vi "Engine Control RT.vi"() -> ()   [LabVIEW 2015]
uses:
  <vilib>/Platform/TimedLoop/XDataNode/timing_clust.ctl
  <vilib>/Platform/TimedLoop/XDataNode/nitl_modes.ctl
  <vilib>/Platform/TimedLoop/XDataNode/wakeup.ctl
  <vilib>/FPGAPlugInAG/cRIO-9118/niLvFpga_Open_cRIO-9118.vi
  <vilib>/rvi/interface/common/dynamic/niFpgaDynamicAddResources.vi
  <vilib>/Utility/error.llb/Error Cluster From Error Code.vi
  <vilib>/rvi/errors/niLvFpgaAdjustHostInterfaceError.vi
  <vilib>/FPGAPlugInAG/Dynamic/niLvFpga_Close_Dynamic.vi
  <vilib>/Platform/TimedLoop/XDataNode/XDataNode.xnode
  <vilib>/rvi/interface/nirviOpenFPGA/nirviOpenFPGA.xnode
  FPGA Bitfiles/EngineControl.lvbitx
  <vilib>/rvi/interface/nirviReadWriteControl/nirviReadWriteControl.xnode
  <vilib>/rvi/interface/nirviCloseFPGA/nirviCloseFPGA.xnode
  <vilib>/Platform/TimedLoop/XDataNode/XDNodeRunTimeDep.lvlib
  <vilib>/rvi/interface/Simulation/niFpgaSimulationCallBeginRW.vi
  NiFpgaLv.dll
panel:
  in  "Tab Control":T1(tab)
  in  "SyncEnable":bool
  in  "SimEnable":bool
  in  "SimSpeed (RPM)":sgl=1000.0
  out "EngineSpeed (RPM)":sgl
  in  "EPTErrorClr":bool
  in  "TDC1 (CAD)":sgl
  out "MAX_CAT":u16=11520
  in  "Stroke (FALSE=2, TRUE=4)":bool=TRUE
  in  "NumberOfCrankTeeth":u16=360
  out "CrankStalled":bool=TRUE
  out "SyncStopped":bool=TRUE
  out "MissedCrankFlag":bool
  out "MissedCamFlag":bool
  out "CrankCount":u16 format="%02.0f"
  out "CAD":sgl format="%05.1f"
  in  "DIControl":T2={"ModuleEnable"=FALSE, "HVEnable"=FALSE, "InjectEnable"=FALSE, "Phase1FirstPeakEnable"=FALSE, "PiezoEnable"=FALSE, "PiezoInvert"=FALSE, "OneShotSelect"=enum."DISABLED", "One Shot Time (msec)"=1.0, "OneShot"=FALSE, "Fault_ClrSig"=FALSE, "HVTarget (V)"=75.0, "Back Boost Time (msec)"=0.25, "DI Scope Trigger Event"=0, "DI Scope Channel 2"=0} {"DI Scope Trigger Event" items=["INJECTION PULSE", "POWER SUPPLY ENABLED"]; "DI Scope Channel 2" items=["INTERNAL HIGH VOLTAGE", "EXTERNAL HIGH VOLTAGE", "BATTERY VOLTAGE"]}
  out "DIData":T3={"ModulePresent"=FALSE, "Module Temperature (C)"=0.0, "Internal High Voltage (V)"=0.0, "External High Voltage (V)"=0.0, "Battery Voltage (V)"=0.0, "Hardware Rev"="\u0000", "Firmware Rev"=0} {"Module Temperature (C)" format="%#.1g"; "Internal High Voltage (V)" format="%#.1f"; "External High Voltage (V)" format="%0#.1g"; "Battery Voltage (V)" format="%#.1g"}
  in  "Channel1 Enable":bool
  out "Critical Faults":T4
  out "Non Critical Faults":T5
  in  "PlsGen_Config":T6={"Window_Start (DBTDC)"=60.0, "Window_End (DBTDC)"=-60.0, "Enable_Inj1"=TRUE, "Duration_Inj1 (msec)"=1.0, "Timing_Inj1 (DBTDC)"=0.0, "Enable_Inj2"=FALSE, "Duration_Inj2 (msec)"=0.0, "Timing_Inj2 (DBTDC)"=0.0, "Enable_Inj3"=FALSE, "Duration_Inj3 (msec)"=0.0, "Timing_Inj3 (DBTDC)"=0.0, "Enable_Inj4"=FALSE, "Duration_Inj4 (msec)"=0.0, "Timing_Inj4 (DBTDC)"=0.0, "Enable_Inj5"=FALSE, "Duration_Inj5 (msec)"=0.0, "Timing_Inj5 (DBTDC)"=0.0}
  in  "DI IPhaseArrayIn":T7(array[cluster])=[{"DriveSrc"=TRUE, "IUpper (A)"=27.0, "ILower (A)"=26.0, "Dur (msec)"=0.3}, {"DriveSrc"=FALSE, "IUpper (A)"=15.0, "ILower (A)"=14.0, "Dur (msec)"=0.0}, {"DriveSrc"=FALSE, "IUpper (A)"=0.0, "ILower (A)"=0.0, "Dur (msec)"=0.0}, {"DriveSrc"=FALSE, "IUpper (A)"=0.0, "ILower (A)"=0.0, "Dur (msec)"=0.0}, {"DriveSrc"=FALSE, "IUpper (A)"=0.0, "ILower (A)"=0.0, "Dur (msec)"=0.0}, {"DriveSrc"=FALSE, "IUpper (A)"=0.0, "ILower (A)"=0.0, "Dur (msec)"=0.0}, {"DriveSrc"=FALSE, "IUpper (A)"=0.0, "ILower (A)"=0.0, "Dur (msec)"=0.0}, {"DriveSrc"=FALSE, "IUpper (A)"=0.0, "ILower (A)"=0.0, "Dur (msec)"=0.0}]
  in  "DIScopeRefresh":bool
  out "DIScope":cluster{sgl, sgl, sgl[][]}(graph)={-3.7e-05, 7.5e-06, array2x4500[9000 elements]}
  out "OLIntegrator":u32
  in  "PFIControl":T8={"ModuleEnable"=FALSE, "LS1Enable"=FALSE, "LS2Enable"=FALSE, "LS3Enable"=FALSE, "LS4Enable"=FALSE, "PFI1Enable"=FALSE, "PFI2Enable"=FALSE, "PFI3Enable"=FALSE, "PFI4Enable"=FALSE, "RecircAlways1"=FALSE, "RecircAlways2"=FALSE, "RecircAlways3"=FALSE, "RecircAlways4"=FALSE, "Phase1FirstPeak1"=FALSE, "Phase1FirstPeak2"=FALSE, "Phase1FirstPeak3"=FALSE, "Phase1FirstPeak4"=FALSE, "OneShotSelect"=enum."DISABLED", "One Shot Time (msec)"=5.0, "OneShot"=FALSE, "Fault_ClrSig"=FALSE}
  in  "PFI IPhaseArrayIn":cluster{"ISetpoint (A)":sgl, "Dur (msec)":sgl}[](array[cluster])=[{"ISetpoint (A)"=4.0, "Dur (msec)"=2.0}, {"ISetpoint (A)"=1.0, "Dur (msec)"=0.0}, {"ISetpoint (A)"=4.0, "Dur (msec)"=2.0}, {"ISetpoint (A)"=1.0, "Dur (msec)"=0.0}, {"ISetpoint (A)"=4.0, "Dur (msec)"=2.0}, {"ISetpoint (A)"=1.0, "Dur (msec)"=0.0}, {"ISetpoint (A)"=4.0, "Dur (msec)"=2.0}, {"ISetpoint (A)"=1.0, "Dur (msec)"=0.0}]
  out "PFIData":T9={"ModulePresent"=FALSE, "Hardware Rev"="\u0000", "Firmware Rev"=0}
  out "Critical Faults 2":T10
  out "Non Critical Faults 2":T11
  in  "LS4Duty":sgl=50.0
  in  "LS3Duty":sgl=50.0
  in  "LS2Duty":sgl=50.0
  in  "LS1Duty":sgl=50.0
  in  "LS4Freq":sgl=5.0
  in  "LS3Freq":sgl=5.0
  in  "LS2Freq":sgl=5.0
  in  "LS1Freq":sgl=5.0
  in  "FuelEnable2":bool
  in  "PFIDuration":sgl=4.0
  in  "CutoffPosition (DBTDC)":sgl=-180.0
  in  "TDC2":sgl=180.0
  in  "FuelTiming (DBTDC)":sgl
  in  "TDC1":sgl
  in  "FuelEnable1":bool
  in  "AfterDuration (msec)":sgl=15.0
  in  "AfterDelay (msec)":sgl=15.0
  in  "MainDuration (msec)":sgl=15.0
  in  "PilotDuration (msec)":sgl=15.0
  in  "PilotAdvance (msec)":sgl=15.0
  in  "AfterEnable1":bool
  in  "PilotEnable1":bool
  in  "MainEnable1":bool
  in  "Cutoff4 (DBTDC)":sgl
  in  "Cutoff3 (DBTDC)":sgl
  in  "Cutoff2 (DBTDC)":sgl
  in  "Cutoff1 (DBTDC)":sgl
  in  "MainSOI (DBTDC)":sgl
  in  "TDC (Absolute CAD)":sgl
  in  "SparkMaxDwell (msec)":sgl=15.0
  in  "SparkMinDwell (msec)":sgl=1.0
  in  "SparkDwell (msec)":sgl=3.0
  in  "SparkCutoffPosition (DBTDC)":sgl=-360.0
  in  "SparkEnd (DBTDC)":sgl
  in  "SparkStart (DBTDC)":sgl
  in  "FuelDuration (msec)":sgl=3.0
  in  "FuelCutoffPosition (DBTDC)":sgl=-360.0
  in  "FuelEnd (DBTDC)":sgl
  in  "FuelStart (DBTDC)":sgl
  in  "SparkActiveLow":bool
  in  "SparkPositionMode (F=End, T=Start)":bool
  in  "SparkEnable":bool
  in  "FuelActiveLow":bool
  in  "FuelPositionMode (F=End, T=Start)":bool
  in  "FuelEnable":bool
  # "http://www.ni.com/powertrain-controls/"
  # "ATTENTION:  The Crank/Cam signals are simulated by the EPT VI.\nHowever, actual signal may be wired to the EPTInSig cluster of the EPT VI in the FPGA.\nRefer to the EPT User manual for details."
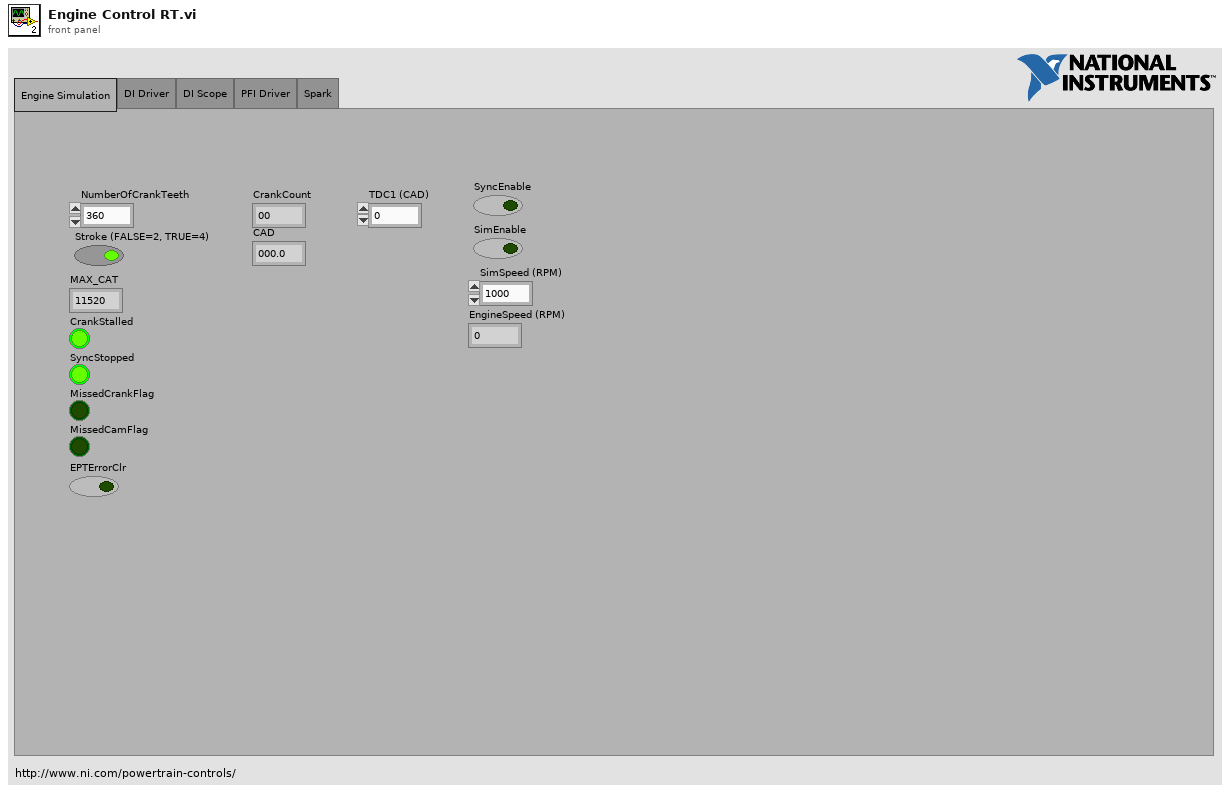
[diagram p1: front panel]
types:
  T1 = enum32{"Engine Simulation", "DI Driver", "DI Scope", "PFI Driver", "Spark"}
  T2 = cluster{"ModuleEnable":bool, "HVEnable":bool, "InjectEnable":bool, "Phase1FirstPeakEnable":bool, "PiezoEnable":bool, "PiezoInvert":bool, "OneShotSelect":enum8{"DISABLED", "CHAN 1", "CHAN 2", "CHAN 3"}, "One Shot Time (msec)":sgl, "OneShot":bool, "Fault_ClrSig":bool, "HVTarget (V)":sgl, "Back Boost Time (msec)":sgl, "DI Scope Trigger Event":u16, "DI Scope Channel 2":u16}
  T3 = cluster{"ModulePresent":bool, "Module Temperature (C)":sgl, "Internal High Voltage (V)":sgl, "External High Voltage (V)":sgl, "Battery Voltage (V)":sgl, "Hardware Rev":string, "Firmware Rev":u8}
  T4 = cluster{"PSCharge":bool, "PSOverLoad":bool, "ShortCircuit":bool, "ModuleTemperature":bool, "HighVoltageDriver":bool, "LowVoltageDriver":bool, "HighVoltageLimit":bool}
  T5 = cluster{"FI1OpenCircuit":bool, "FI2OpenCircuit":bool, "FI3OpenCircuit":bool}
  T6 = cluster{"Window_Start (DBTDC)":sgl, "Window_End (DBTDC)":sgl, "Enable_Inj1":bool, "Duration_Inj1 (msec)":sgl, "Timing_Inj1 (DBTDC)":sgl, "Enable_Inj2":bool, "Duration_Inj2 (msec)":sgl, "Timing_Inj2 (DBTDC)":sgl, "Enable_Inj3":bool, "Duration_Inj3 (msec)":sgl, "Timing_Inj3 (DBTDC)":sgl, "Enable_Inj4":bool, "Duration_Inj4 (msec)":sgl, "Timing_Inj4 (DBTDC)":sgl, "Enable_Inj5":bool, "Duration_Inj5 (msec)":sgl, "Timing_Inj5 (DBTDC)":sgl}
  T7 = cluster{"DriveSrc":bool, "IUpper (A)":sgl, "ILower (A)":sgl, "Dur (msec)":sgl}[]
  T8 = cluster{"ModuleEnable":bool, "LS1Enable":bool, "LS2Enable":bool, "LS3Enable":bool, "LS4Enable":bool, "PFI1Enable":bool, "PFI2Enable":bool, "PFI3Enable":bool, "PFI4Enable":bool, "RecircAlways1":bool, "RecircAlways2":bool, "RecircAlways3":bool, "RecircAlways4":bool, "Phase1FirstPeak1":bool, "Phase1FirstPeak2":bool, "Phase1FirstPeak3":bool, "Phase1FirstPeak4":bool, "OneShotSelect":enum8{"DISABLED", "PFI 1", "PFI 2", "PFI 3", "PFI 4"}, "One Shot Time (msec)":sgl, "OneShot":bool, "Fault_ClrSig":bool}
  T9 = cluster{"ModulePresent":bool, "Hardware Rev":string, "Firmware Rev":u8}
  T10 = cluster{"LS1Short":bool, "LS2Short":bool, "LS3Short":bool, "LS4Short":bool, "PFI1Short":bool, "PFI2Short":bool, "PFI3Short":bool, "PFI4Short":bool}
  T11 = cluster{"LS1Open":bool, "LS2Open":bool, "LS3Open":bool, "LS4Open":bool, "PFI1Open":bool, "PFI2Open":bool, "PFI3Open":bool, "PFI4Open":bool}
  T12 = typedef "XDNodeRunTimeDep.lvlib/timing_clust.ctl" = cluster{"Expected End [f-1]":u64, "Actual End [f-1]":u64, "Finished Late? [f-1]":bool, "Expected End [i-1]":u64, "Actual End [i-1]":u64, "Finished Late? [i-1]":bool, "Expected Start [i]":u64, "Actual Start [i]":u64, "Expected Start [f]":u64, "Actual Start [f]":u64, "Source Name":string, "Structure Name":string, "Period":i64, "Deadline":i64, "Offset":i64, "Start":i64, "Priority":i32, "Timeout":i32, "Mode":T13, "Wakeup Reason":T14, "Error":errorcluster, "Source Type":string, "Secondary Source Type":string, "Global End Time":u64, "Global Start Time":u64, "Frame Duration":u64, "Iteration Duration":u64, "Assigned CPU":i32, "I/O Scan Engine Mode":u32}
  T13 = typedef "XDNodeRunTimeDep.lvlib/nitl_modes.ctl" = enum32{"No Change", "Process missed periods, maintain original phase", "Discard missed periods, maintain original phase", "Process missed periods, ignore original phase", "Discard missed periods, ignore original phase"}
  T14 = typedef "XDNodeRunTimeDep.lvlib/wakeup.ctl" = enum32{"Normal", "Aborted", "Asynchronous wakeup", "Timing source error", "Timed loop error", "Timeout"}
  T15 = cluster{"MainEnable1":bool, "PilotEnable1":bool, "PreEnable1":bool, "AfterEnable1":bool, "PostEnable1":bool, "MainStartPosition1":u16, "PilotAdvance1":u32, "PilotDuration1":u32, "PreAdvance1":u32, "PreDuration1":u32, "MainDuration1":u32, "AfterDelay1":u32, "AfterDuration1":u32, "PostDelay1":u32, "PostDuration1":u32, "CutoffPosition1":u16}
  T16 = cluster{"SparkEnable":bool, "PositionMode":bool, "ActiveLow":bool, "StartPosition":u16, "EndPosition":u16, "CutoffPosition":u16, "Dwell":u32, "MinDwell":u32, "MaxDwell":u32}
  T17 = cluster{"FuelEnable":bool, "PositionMode":bool, "ActiveLow":bool, "StartPosition":u16, "EndPosition":u16, "CutoffPosition":u16, "Duration":u32}
  T18 = cluster{"Element":u32, "Timed Out?":bool, "Elements Left":u32}
  T19 = cluster{"NumberOfCrankTeeth":u16, "Stroke (FALSE=2, TRUE=4)":bool, "CrankStallPeriod":u32, "CrankCountStart":u16, "PeriodAccumCount":u16, "SyncEnable":bool, "SimEnable":bool, "MissedCrankFlagClr":bool, "MissedCamFlagClr":bool, "SimPeriod":u32, "WatchdogIn":bool}
  T20 = cluster{"ModulePresent":bool, "LVSense":u8, "HVSense":u8, "HVSense2":u8, "TempSense":i8, "Fault1":u8, "Fault2":u8, "OLIntegrator":u32, "HardwareRev":u8, "FirmwareRev":u8}
  T21 = cluster{"CrankSigOS":bool, "CrankStalled":bool, "SyncStopped":bool, "MissedCrankFlag":bool, "MissedCamFlag":bool, "Period":u32, "PeriodAccum":u32, "CrankCount":u16, "CurrentPosition":u16, "MAX_CAT":u16}
  T22 = cluster{"Channel Enable":bool, "Window_Start":u16, "Window_End":u16, "Enable_Inj1":bool, "Duration_Inj1":u32, "Timing_Inj1":u16, "Enable_Inj2":bool, "Duration_Inj2":u32, "Timing_Inj2":u16, "Enable_Inj3":bool, "Duration_Inj3":u32, "Timing_Inj3":u16, "Enable_Inj4":bool, "Duration_Inj4":u32, "Timing_Inj4":u16, "Enable_Inj5":bool, "Duration_Inj5":u32, "Timing_Inj5":u16}
  T23 = cluster{"ModuleEnable":bool, "WatchdogIn":bool, "OneShotSelect":enum8{"DISABLED", "CHAN 1", "CHAN 2", "CHAN 3"}, "OneShotTime":u32, "OneShot":bool, "Control":u8, "Control2":u8, "HostMode":u8, "HostCommand":u32, "HVTarget":u8, "BackBoostTime":u8, "Fault_ClrSig":bool}
  T24 = cluster{"IPhaseDrive (TRUE=HV, FALSE=LV)":bool, "IPhaseCurrentUpper":u16, "IPhaseCurrentLower":u16, "IPhaseDuration":u16}[]
  T25 = cluster{"LS1Period":u32, "LS1PulseWidth":u32, "LS2Period":u32, "LS2PulseWidth":u32, "LS3Period":u32, "LS3PulseWidth":u32, "LS4Period":u32, "LS4PulseWidth":u32}
  T26 = cluster{"ModulePresent":bool, "Fault1":u8, "Fault2":u8, "HardwareRev":u8, "FirmwareRev":u8}
  T27 = cluster{"IPhaseCurrent":u16, "IPhaseDuration":u16}[]
  T28 = cluster{"ModuleEnable":bool, "WatchdogIn":bool, "OneShotSelect":enum8{"DISABLED", "PFI 1", "PFI 2", "PFI 3", "PFI 4"}, "OneShotTime":u32, "OneShot":bool, "Control":u16, "HostMode":u8, "HostCommand":u32, "Fault_ClrSig":bool}
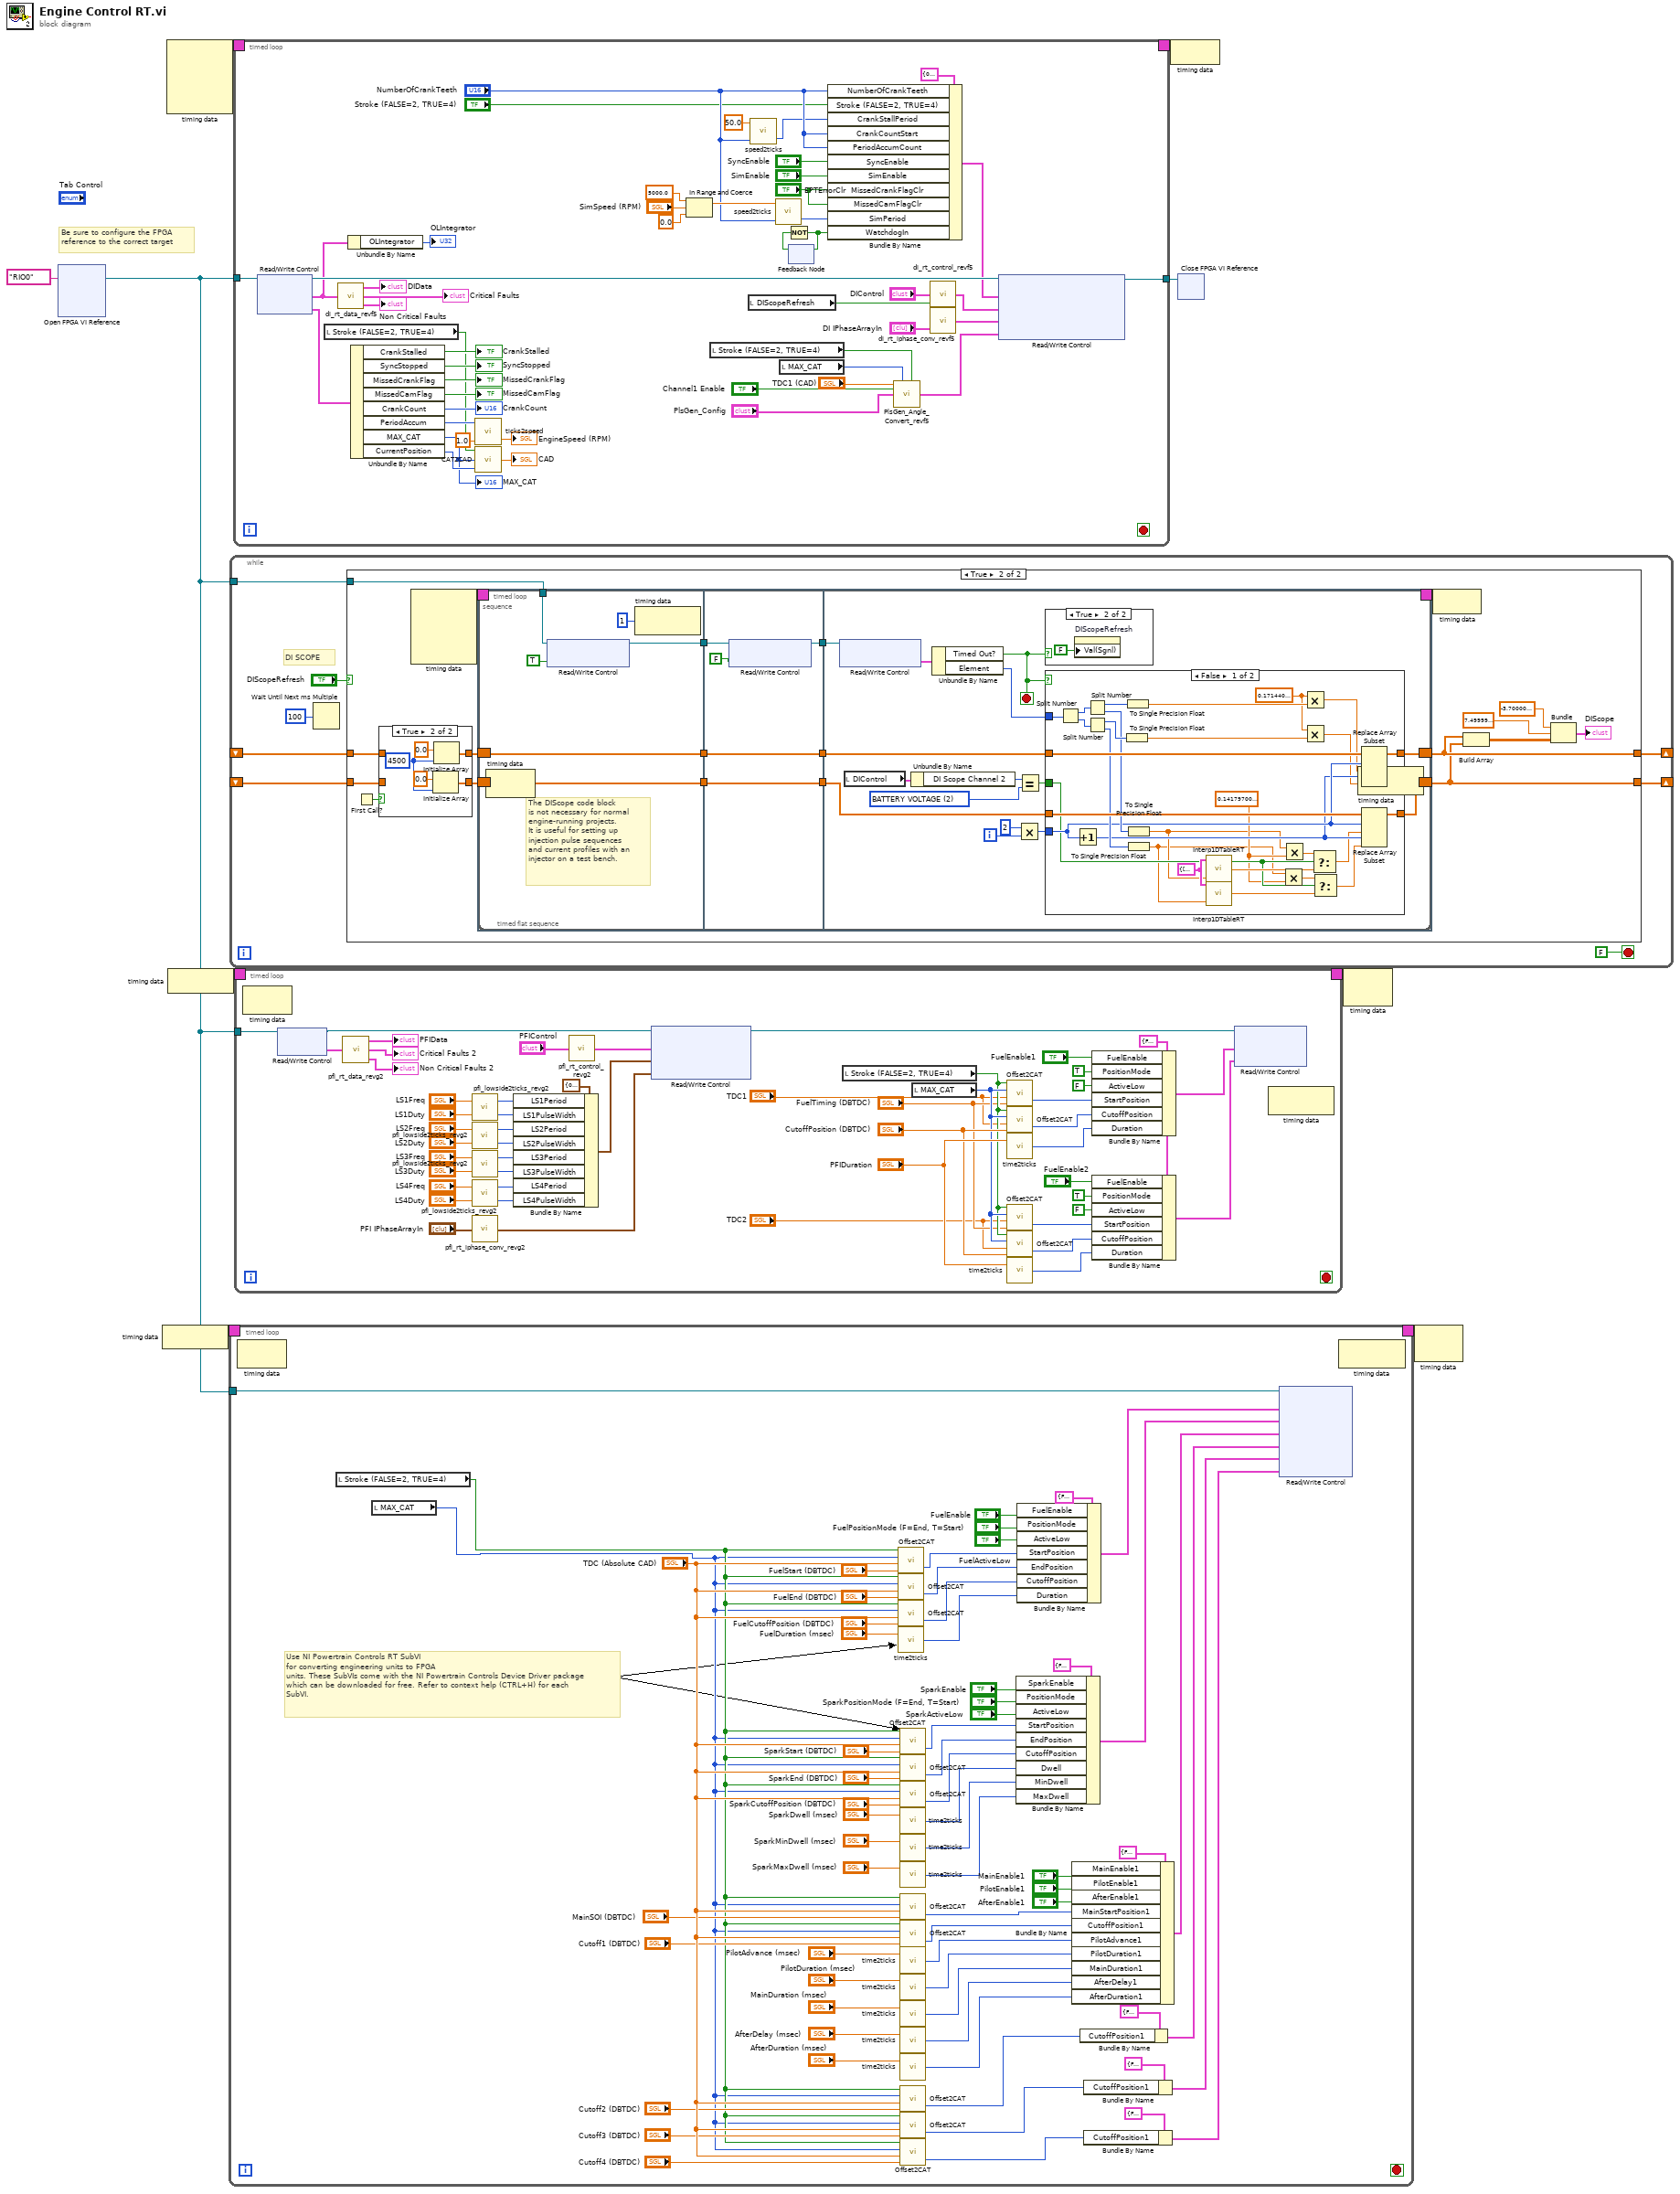
[diagram p0: block diagram]
diagram:
  # "Be sure to configure the FPGA\nreference to the correct target"
  n1 = xnode "Open FPGA VI Reference"("resource name"=tag "RIO0") -> ("FPGA VI Reference Out"=w2:refnum<k20>)  [unwired: 1 in, 1 out]
  n2 = node-c288() -> (w4:T12)
  n3 = node-c288() -> (w9:T12)  [unwired: 4 in]
  n4 = node-c288() -> (w6:T12)
  n5 = timed-loop {
    timing: w4 -> [_]
    timing-out: [_] -> w3
    tunnel: w2 -> [w16]
    stop <- _ stop-if-true
    # "Use NI Powertrain Controls RT SubVI\nfor converting engineering units to FPGA\nunits. These SubVIs come with the NI Powertrain Controls Device Driver package which can be downloaded for free. Refer to context help (CTRL+H) for each\nSubVI."
    n6 = node-c288() -> ()  [unwired: 1 in, 1 out]
    n7 = local read "Stroke (FALSE=2, TRUE=4)"() -> (w19:bool)
    n8 = local read "MAX_CAT"() -> (w18:u16)
    n9 = call <vilib>:"Offset2CAT.vi"("Offset (CAD Before TDC)"="FuelStart (DBTDC)", "TDC (Absolute CAD)"="TDC (Absolute CAD)", "MAX_CAT"=w18, "Stroke (FALSE=2, TRUE=4)"=w19) -> ("CAT"=w28:u16)  [unwired: 1 out]
    n10 = call <vilib>:"Offset2CAT.vi"("Offset (CAD Before TDC)"="FuelEnd (DBTDC)", "TDC (Absolute CAD)"="TDC (Absolute CAD)", "MAX_CAT"=w18, "Stroke (FALSE=2, TRUE=4)"=w19) -> ("CAT"=w30:u16)  [unwired: 1 out]
    n11 = call <vilib>:"Offset2CAT.vi"("Offset (CAD Before TDC)"="FuelCutoffPosition (DBTDC)", "TDC (Absolute CAD)"="TDC (Absolute CAD)", "MAX_CAT"=w18, "Stroke (FALSE=2, TRUE=4)"=w19) -> ("CAT"=w32:u16)  [unwired: 1 out]
    n12 = call <vilib>:"time2ticks.vi"("Time (msec)"="FuelDuration (msec)") -> ("Ticks"=w33:u32)  [unwired: 1 in]
    n13 = call <vilib>:"Offset2CAT.vi"("Offset (CAD Before TDC)"="SparkStart (DBTDC)", "TDC (Absolute CAD)"="TDC (Absolute CAD)", "MAX_CAT"=w18, "Stroke (FALSE=2, TRUE=4)"=w19) -> ("CAT"=w39:u16)  [unwired: 1 out]
    n14 = call <vilib>:"Offset2CAT.vi"("Offset (CAD Before TDC)"="SparkEnd (DBTDC)", "TDC (Absolute CAD)"="TDC (Absolute CAD)", "MAX_CAT"=w18, "Stroke (FALSE=2, TRUE=4)"=w19) -> ("CAT"=w40:u16)  [unwired: 1 out]
    n15 = call <vilib>:"Offset2CAT.vi"("Offset (CAD Before TDC)"="SparkCutoffPosition (DBTDC)", "TDC (Absolute CAD)"="TDC (Absolute CAD)", "MAX_CAT"=w18, "Stroke (FALSE=2, TRUE=4)"=w19) -> ("CAT"=w41:u16)  [unwired: 1 out]
    n16 = call <vilib>:"time2ticks.vi"("Time (msec)"="SparkDwell (msec)") -> ("Ticks"=w42:u32)  [unwired: 1 in]
    n17 = call <vilib>:"time2ticks.vi"("Time (msec)"="SparkMinDwell (msec)") -> ("Ticks"=w45:u32)  [unwired: 1 in]
    n18 = call <vilib>:"time2ticks.vi"("Time (msec)"="SparkMaxDwell (msec)") -> ("Ticks"=w46:u32)  [unwired: 1 in]
    n19 = call <vilib>:"Offset2CAT.vi"("Offset (CAD Before TDC)"="MainSOI (DBTDC)", "TDC (Absolute CAD)"="TDC (Absolute CAD)", "MAX_CAT"=w18, "Stroke (FALSE=2, TRUE=4)"=w19) -> ("CAT"=w57:u16)  [unwired: 1 out]
    n20 = call <vilib>:"Offset2CAT.vi"("Offset (CAD Before TDC)"="Cutoff1 (DBTDC)", "TDC (Absolute CAD)"="TDC (Absolute CAD)", "MAX_CAT"=w18, "Stroke (FALSE=2, TRUE=4)"=w19) -> ("CAT"=w58:u16)  [unwired: 1 out]
    n21 = call <vilib>:"time2ticks.vi"("Time (msec)"="PilotAdvance (msec)") -> ("Ticks"=w64:u32)  [unwired: 1 in]
    n22 = call <vilib>:"time2ticks.vi"("Time (msec)"="PilotDuration (msec)") -> ("Ticks"=w65:u32)  [unwired: 1 in]
    n23 = call <vilib>:"time2ticks.vi"("Time (msec)"="MainDuration (msec)") -> ("Ticks"=w66:u32)  [unwired: 1 in]
    n24 = call <vilib>:"time2ticks.vi"("Time (msec)"="AfterDelay (msec)") -> ("Ticks"=w67:u32)  [unwired: 1 in]
    n25 = call <vilib>:"time2ticks.vi"("Time (msec)"="AfterDuration (msec)") -> ("Ticks"=w68:u32)  [unwired: 1 in]
    n26 = call <vilib>:"Offset2CAT.vi"("Offset (CAD Before TDC)"="Cutoff2 (DBTDC)", "TDC (Absolute CAD)"="TDC (Absolute CAD)", "MAX_CAT"=w18, "Stroke (FALSE=2, TRUE=4)"=w19) -> ("CAT"=w72:u16)  [unwired: 1 out]
    n27 = call <vilib>:"Offset2CAT.vi"("Offset (CAD Before TDC)"="Cutoff3 (DBTDC)", "TDC (Absolute CAD)"="TDC (Absolute CAD)", "MAX_CAT"=w18, "Stroke (FALSE=2, TRUE=4)"=w19) -> ("CAT"=w73:u16)  [unwired: 1 out]
    n28 = call <vilib>:"Offset2CAT.vi"("Offset (CAD Before TDC)"="Cutoff4 (DBTDC)", "TDC (Absolute CAD)"="TDC (Absolute CAD)", "MAX_CAT"=w18, "Stroke (FALSE=2, TRUE=4)"=w19) -> ("CAT"=w74:u16)  [unwired: 1 out]
    n29 = Bundle By Name(cluster=T16 {"SparkEnable"=FALSE, "PositionMode"=FALSE, "ActiveLow"=FALSE, "StartPosition"=0, "EndPosition"=0, "CutoffPosition"=0, "Dwell"=0, "MinDwell"=0, "MaxDwell"=0} ("SparkControl"), "SparkEnable"="SparkEnable", "PositionMode"="SparkPositionMode (F=End, T=Start)", "ActiveLow"="SparkActiveLow", "StartPosition"=w39, "EndPosition"=w40, "CutoffPosition"=w41, "Dwell"=w42, "MinDwell"=w45, "MaxDwell"=w46) -> (w14:T16)
    n30 = Bundle By Name(cluster=T17 {"FuelEnable"=FALSE, "PositionMode"=FALSE, "ActiveLow"=FALSE, "StartPosition"=0, "EndPosition"=0, "CutoffPosition"=0, "Duration"=0} ("FuelControl"), "FuelEnable"="FuelEnable", "PositionMode"="FuelPositionMode (F=End, T=Start)", "ActiveLow"="FuelActiveLow", "StartPosition"=w28, "EndPosition"=w30, "CutoffPosition"=w32, "Duration"=w33) -> (w15:T17)
    n31 = Bundle By Name(cluster=T15 {"MainEnable1"=FALSE, "PilotEnable1"=FALSE, "PreEnable1"=FALSE, "AfterEnable1"=FALSE, "PostEnable1"=FALSE, "MainStartPosition1"=0, "PilotAdvance1"=0, "PilotDuration1"=0, "PreAdvance1"=0, "PreDuration1"=0, "MainDuration1"=0, "AfterDelay1"=0, "AfterDuration1"=0, "PostDelay1"=0, "PostDuration1"=0, "CutoffPosition1"=0} ("MPControl1"), "MainEnable1"="MainEnable1", "PilotEnable1"="PilotEnable1", "AfterEnable1"="AfterEnable1", "MainStartPosition1"=w57, "CutoffPosition1"=w58, "PilotAdvance1"=w64, "PilotDuration1"=w65, "MainDuration1"=w66, "AfterDelay1"=w67, "AfterDuration1"=w68) -> (w10:T15)
    n32 = Bundle By Name(cluster=T15 {"MainEnable1"=FALSE, "PilotEnable1"=FALSE, "PreEnable1"=FALSE, "AfterEnable1"=FALSE, "PostEnable1"=FALSE, "MainStartPosition1"=0, "PilotAdvance1"=0, "PilotDuration1"=0, "PreAdvance1"=0, "PreDuration1"=0, "MainDuration1"=0, "AfterDelay1"=0, "AfterDuration1"=0, "PostDelay1"=0, "PostDuration1"=0, "CutoffPosition1"=0} ("MPControl1"), "CutoffPosition1"=w72) -> (w11:T15)
    n33 = Bundle By Name(cluster=T15 {"MainEnable1"=FALSE, "PilotEnable1"=FALSE, "PreEnable1"=FALSE, "AfterEnable1"=FALSE, "PostEnable1"=FALSE, "MainStartPosition1"=0, "PilotAdvance1"=0, "PilotDuration1"=0, "PreAdvance1"=0, "PreDuration1"=0, "MainDuration1"=0, "AfterDelay1"=0, "AfterDuration1"=0, "PostDelay1"=0, "PostDuration1"=0, "CutoffPosition1"=0} ("MPControl1"), "CutoffPosition1"=w73) -> (w12:T15)
    n34 = Bundle By Name(cluster=T15 {"MainEnable1"=FALSE, "PilotEnable1"=FALSE, "PreEnable1"=FALSE, "AfterEnable1"=FALSE, "PostEnable1"=FALSE, "MainStartPosition1"=0, "PilotAdvance1"=0, "PilotDuration1"=0, "PreAdvance1"=0, "PreDuration1"=0, "MainDuration1"=0, "AfterDelay1"=0, "AfterDuration1"=0, "PostDelay1"=0, "PostDuration1"=0, "CutoffPosition1"=0} ("MPControl1"), "CutoffPosition1"=w74) -> (w13:T15)
    n35 = xnode "Read/Write Control"("FPGA VI Reference In"=w16, "FuelControl"=w15, "SparkControl"=w14, "MPControl1"=w10, "MPControl2"=w11, "MPControl3"=w12, "MPControl4"=w13) -> ()  [unwired: 1 in, 2 out]
    n36 = node-c288() -> ()  [unwired: 1 in, 1 out]
  }
  n37 = while {
    shift-right: [w82] -> _
    shift-left: _ -> [w84]
    shift-right: [w81] -> _
    shift-left: _ -> [w83]
    tunnel: w2 -> [w78]
    stop <- FALSE stop-if-true
    # "DI SCOPE"
    n38 = Wait Until Next ms Multiple(millisecond multiple=u32 100) -> ()  [unwired: 1 out]
    n39 = case shown="True" "DIScopeRefresh" {
      tunnel: w84 -> [w86 w98]
      tunnel: w83 -> [w85 w97]
      tunnel: [w86 w96] -> w82
      tunnel: [w85 w92] -> w81
      tunnel: w78 -> [_ w87]
      frame False {
      }
      frame True {
        n40 = First Call?() -> (First Call?: T/F=w100:bool)
        n41 = case shown="True" w100 {
          tunnel: [w188 w192] -> w99
          tunnel: [w187 w191] -> w95
          tunnel: w98 -> [w188 _]
          tunnel: w97 -> [w187 _]
          frame False {
          }
          frame True {
            w189 = 4500 ("dimension size")
            n42 = Initialize Array(sgl 0.0 ("element"), w189) -> (w191:sgl[])
            n43 = Initialize Array(sgl 0.0 ("element"), w189) -> (w192:sgl[])
          }
        }
        n44 = node-c288() -> (w94:T12)  [unwired: 4 in]
        n45 = timed-loop "Timed Loop" {
          shift-right: [w103] -> w96
          shift-left: w99 -> [w104]
          shift-right: [w101] -> w92
          shift-left: w95 -> [w102]
          tunnel: w87 -> [w105]
          timing: w94 -> [_]
          timing-out: [_] -> w93
          i -> [w138]
          stop <- w134 stop-if-true
          n46 = timed-sequence {
            timing: _ -> [_]
            timing-out: _ -> [_]
            tunnel: w105 -> [w116]
            tunnel: w104 -> [w115]
            tunnel: [w114] -> w103
            tunnel: w102 -> [w113]
            tunnel: [w112] -> w101
            n47 = timed-flat-sequence {
              tunnel: w113 -> [w121]
              tunnel: w115 -> [w122]
              tunnel: w116 -> [w118]
              tunnel: [w122] -> w109
              tunnel: [w121] -> w108
              tunnel: [w119] -> w107
              tunnel: [w131] -> w111
              tunnel: [w130] -> w110
              tunnel: w107 -> [w128]
              tunnel: w108 -> [w130]
              tunnel: w109 -> [w131]
              tunnel: [w127] -> w106
              tunnel: [w145] -> w114
              tunnel: [w144] -> w112
              tunnel: w111 -> [w148]
              tunnel: w110 -> [w147]
              tunnel: w106 -> [w140]
              frame #0 {
                # "The DIScope code block\nis not necessary for normal\nengine-running projects.\nIt is useful for setting up\ninjection pulse sequences\nand current profiles with an\ninjector on a test bench."
                n48 = xnode "Read/Write Control"("FPGA VI Reference In"=w118, "DI1_ScopeRead"=TRUE ("DIScopeRead")) -> ("FPGA VI Reference Out"=w119:refnum<k20>)  [unwired: 1 in, 1 out]
                n49 = node-c288(i64 1 ("Start")) -> ()  [unwired: 1 out]
              }
              frame #1 {
                n50 = xnode "Read/Write Control"("FPGA VI Reference In"=w128, "DI1_ScopeRead"=FALSE ("DIScopeRead")) -> ("FPGA VI Reference Out"=w127:refnum<k20>)  [unwired: 1 in, 1 out]
              }
              frame #2 {
                w143 = u16 2 items=["INTERNAL HIGH VOLTAGE", "EXTERNAL HIGH VOLTAGE", "BATTERY VOLTAGE"] ("DI Scope Channel 2")
                n51 = xnode "Read/Write Control"("FPGA VI Reference In"=w140) -> ("DI1_ScopeData"=w141:T18)  [unwired: 1 in, 2 out]
                n52 = local read "DIControl"() -> (w137:T2)
                n53 = Unbundle By Name(w137) -> ("DI Scope Channel 2"=w136:u16)
                n54 = Unbundle By Name(w141) -> ("Timed Out?"=w134:bool, "Element"=w135:u32)
                n55 = Multiply(x=2, y=w138) -> (x*y=w139:i32)
                n56 = Equal?(x=w136, y=w143) -> (x = y?=w142:bool)
                n57 = case shown="True" w134 {
                  frame False {
                  }
                  frame True {
                    n58 = property on="DIScopeRefresh" class="Bool (strict)"("Val(Sgnl)"=FALSE ("Value (Signaling)")) -> ()  [unwired: 2 in, 2 out]
                  }
                }
                n59 = case shown="False" w134 {
                  tunnel: w135 -> [w178 _]
                  tunnel: w148 -> [w175 w180]
                  tunnel: w147 -> [w174 w179]
                  tunnel: w139 -> [w167 _]
                  tunnel: [w169 w180] -> w145
                  tunnel: [w168 w179] -> w144
                  tunnel: w142 -> [w163 _]
                  frame False {
                    w160 = sgl 0.17144 ("y")
                    w165 = cluster{"Counts (8bit)":sgl[], "Volts":sgl[]} {"Counts (8bit)"=[0.0, 26.0, 50.0, 74.0, 97.0, 120.0, 144.0, 167.0, 190.0, 213.0, 237.0], "Volts"=[0.0, 20.0, 40.0, 60.0, 80.0, 100.0, 120.0, 140.0, 160.0, 180.0, 200.0]} ("HVTable")
                    w152 = sgl 0.141797 ("y")
                    n60 = Split Number(x=w178) -> (hi(x)=w177:u16, lo(x)=w176:u16)
                    n61 = Increment(x=w167) -> (x+1=w166:i32)
                    n62 = Split Number(x=w177) -> (hi(x)=w171:u8, lo(x)=w170:u8)
                    n63 = Split Number(x=w176) -> (hi(x)=w173:u8, lo(x)=w172:u8)
                    n64 = To Single Precision Float(number=w173) -> (single precision float=w159:sgl)
                    n65 = To Single Precision Float(number=w171) -> (single precision float=w161:sgl)
                    n66 = To Single Precision Float(number=w170) -> (single precision float=w151:sgl)
                    n67 = To Single Precision Float(number=w172) -> (single precision float=w150:sgl)
                    n68 = call <vilib>:"Interp1DTableRT.vi"("X"=w151, "1DTable"=w165) -> ("Y"=w164:sgl)  [unwired: 1 in]
                    n69 = call <vilib>:"Interp1DTableRT.vi"("X"=w150, "1DTable"=w165) -> ("Y"=w162:sgl)  [unwired: 1 in]
                    n70 = Multiply(x=w150, y=w152) -> (x*y=w154:sgl)
                    n71 = Multiply(x=w151, y=w152) -> (x*y=w153:sgl)
                    n72 = Multiply(x=w160, y=w161) -> (x*y=w157:sgl)
                    n73 = Multiply(x=w160, y=w159) -> (x*y=w158:sgl)
                    n74 = Select(t=w153, s=w163, f=w164) -> (s? t:f=w155:sgl)
                    n75 = Select(t=w154, s=w163, f=w162) -> (s? t:f=w156:sgl)
                    n76 = Replace Array Subset(array=w175, new element #1=w157, index #1=w167, new element #2=w158, index #2=w166) -> (w169:sgl[])
                    n77 = Replace Array Subset(array=w174, new element #1=w155, index #1=w167, new element #2=w156, index #2=w166) -> (w168:sgl[])
                  }
                  frame True {
                  }
                }
              }
            }
          }
          n78 = node-c288() -> ()  [unwired: 1 in, 1 out]
          n79 = node-c288() -> ()  [unwired: 1 in, 1 out]
        }
        n80 = node-c288(w93) -> ()
        n81 = Build Array(w96, w92) -> (w89:sgl[][])
        n82 = Bundle("Offset"=sgl -3.7e-05, "Scale"=sgl 7.5e-06, w89) -> (→"DIScope":cluster{"Offset":sgl, "Scale":sgl, sgl[][]})  [unwired: 1 out]
      }
    }
  }
  n83 = timed-loop {
    timing: w9 -> [_]
    timing-out: [_] -> w8
    tunnel: w2 -> [w239]
    tunnel: [w240] -> w7
    stop <- _ stop-if-true
    n84 = xnode "Read/Write Control"("FPGA VI Reference In"=w239) -> ("FPGA VI Reference Out"=w241:refnum<k20>, "DI1_Data"=w200:T20, "EPTData"=w203:T21)  [unwired: 1 in, 1 out]
    n85 = local read "Stroke (FALSE=2, TRUE=4)"() -> (w206:bool)
    n86 = call <vilib>:"di_rt_data_revf5.vi"("DIDataFromFPGA"=w200) -> ("Non Critical Faults"=→"Non Critical Faults":T5, "Critical Faults"=→"Critical Faults":T4, "DIData"=→"DIData":T3)  [unwired: 2 in]
    n87 = Unbundle By Name(w200) -> ("OLIntegrator"=→"OLIntegrator":u32)
    n88 = Unbundle By Name(w203) -> ("CrankStalled"=→"CrankStalled":bool, "SyncStopped"=→"SyncStopped":bool, "MissedCrankFlag"=→"MissedCrankFlag":bool, "MissedCamFlag"=→"MissedCamFlag":bool, "CrankCount"=→"CrankCount":u16, "PeriodAccum"=w208:u32, "MAX_CAT"=w204:u16, "CurrentPosition"=w207:u16)
    "MAX_CAT" <- w204
    n89 = call <vilib>:"ticks2speed.vi"("PulsesPerRotation"=sgl 1.0, "Period (ticks)"=w208) -> ("Speed (RPM)"=→"EngineSpeed (RPM)":sgl)  [unwired: 1 in, 1 out]
    n90 = call <vilib>:"CAT2CAD.vi"("CAT"=w207, "MAX_CAT"=w204, "Stroke (FALSE=2, TRUE=4)"=w206) -> ("CAD"=→"CAD":sgl)
    n91 = In Range and Coerce(upper limit=sgl 5000.0, x="SimSpeed (RPM)", lower limit=sgl 0.0) -> (coerced(x)=w234:sgl)  [unwired: 1 out]
    n92 = local read "Stroke (FALSE=2, TRUE=4)"() -> (w218:bool)
    n93 = local read "DIScopeRefresh"() -> (w238:bool)
    n94 = call <vilib>:"speed2ticks.vi"("PulsesPerRotation"="NumberOfCrankTeeth", "Speed (RPM)"=sgl 50.0) -> ("Period (ticks)"=w226:u32)  [unwired: 1 in, 1 out]
    n95 = call <vilib>:"speed2ticks.vi"("PulsesPerRotation"="NumberOfCrankTeeth", "Speed (RPM)"=w234) -> ("Period (ticks)"=w231:u32)  [unwired: 1 in, 1 out]
    n96 = local read "MAX_CAT"() -> (w217:u16)
    n97 = feedback #1() -> (w223:bool)  [unwired: 1 in]
    n98 = Not(x=w223) -> (.not. x?=w222:bool)
    n99 = feedback-in #1(w222) -> ()
    n100 = Bundle By Name(cluster=T19 {"NumberOfCrankTeeth"=0, "Stroke (FALSE=2, TRUE=4)"=FALSE, "CrankStallPeriod"=0, "CrankCountStart"=0, "PeriodAccumCount"=0, "SyncEnable"=FALSE, "SimEnable"=FALSE, "MissedCrankFlagClr"=FALSE, "MissedCamFlagClr"=FALSE, "SimPeriod"=0, "WatchdogIn"=FALSE} ("EPTControl"), "NumberOfCrankTeeth"="NumberOfCrankTeeth", "Stroke (FALSE=2, TRUE=4)"="Stroke (FALSE=2, TRUE=4)", "CrankStallPeriod"=w226, "CrankCountStart"="NumberOfCrankTeeth", "PeriodAccumCount"="NumberOfCrankTeeth", "SyncEnable"="SyncEnable", "SimEnable"="SimEnable", "MissedCrankFlagClr"="EPTErrorClr", "MissedCamFlagClr"="EPTErrorClr", "SimPeriod"=w231, "WatchdogIn"=w222) -> (w221:T19)
    n101 = call <vilib>:"PlsGen_Angle_Convert_revf5.vi"("TDC (Absolute CAD)"="TDC1 (CAD)", "MAX_CAT"=w217, "Stroke (FALSE=2, TRUE=4)"=w218, "Channel Enable"="Channel1 Enable", "PlsGen_Angle_Config_In"="PlsGen_Config") -> ("PlsGen_Config_Out"=w220:T22)  [unwired: 10 in]
    n102 = call <vilib>:"di_rt_control_revf5.vi"("DIScopeTransfer"=w238, "DIControl"="DIControl") -> ("DIControlToFPGA"=w237:T23)  [unwired: 3 in]
    n103 = call <vilib>:"di_rt_iphase_conv_revf5.vi"("IPhaseArrayIn"="DI IPhaseArrayIn") -> ("IPhaseArrayOut"=w197:T24)
    n104 = xnode "Read/Write Control"("FPGA VI Reference In"=w241, "EPTControl"=w221, "DI1_Control"=w237, "DI1_IPhaseInterface"=w197, "PlsGen_Config_Channel1"=w220) -> ("FPGA VI Reference Out"=w240:refnum<k20>)  [unwired: 1 in, 1 out]
  }
  n105 = timed-loop {
    timing: w6 -> [_]
    timing-out: [_] -> w5
    tunnel: w2 -> [w290]
    stop <- _ stop-if-true
    w266 = T17 {"FuelEnable"=FALSE, "PositionMode"=FALSE, "ActiveLow"=FALSE, "StartPosition"=0, "EndPosition"=0, "CutoffPosition"=0, "Duration"=0} ("FuelControlGlobal")
    n106 = node-c288() -> ()  [unwired: 1 in, 1 out]
    n107 = xnode "Read/Write Control"("FPGA VI Reference In"=w290) -> ("FPGA VI Reference Out"=w244:refnum<k20>, "PFIData"=w294:T26)  [unwired: 1 in, 1 out]
    n108 = call <vilib>:"pfi_rt_data_revg2.vi"("PFIDataFromFPGA"=w294) -> ("Non Critical Faults"=→"Non Critical Faults 2":T11, "Critical Faults"=→"Critical Faults 2":T10, "PFIData"=→"PFIData":T9)  [unwired: 2 in]
    n109 = call <vilib>:"pfi_lowside2ticks_revg2.vi"("DutyCycle (%)"="LS1Duty", "Frequency (Hz)"="LS1Freq") -> ("LSPulseWidthTicks"=w283:u32, "LSPeriodTicks"=w282:u32)
    n110 = call <vilib>:"pfi_lowside2ticks_revg2.vi"("DutyCycle (%)"="LS2Duty", "Frequency (Hz)"="LS2Freq") -> ("LSPulseWidthTicks"=w285:u32, "LSPeriodTicks"=w284:u32)
    n111 = call <vilib>:"pfi_lowside2ticks_revg2.vi"("DutyCycle (%)"="LS3Duty", "Frequency (Hz)"="LS3Freq") -> ("LSPulseWidthTicks"=w287:u32, "LSPeriodTicks"=w286:u32)
    n112 = call <vilib>:"pfi_lowside2ticks_revg2.vi"("DutyCycle (%)"="LS4Duty", "Frequency (Hz)"="LS4Freq") -> ("LSPulseWidthTicks"=w289:u32, "LSPeriodTicks"=w288:u32)
    n113 = call <vilib>:"pfi_rt_iphase_conv_revg2.vi"("IPhaseArrayIn"="PFI IPhaseArrayIn") -> ("IPhaseArrayOut"=w246:T27)
    n114 = Bundle By Name(cluster=T25 {"LS1Period"=0, "LS1PulseWidth"=0, "LS2Period"=0, "LS2PulseWidth"=0, "LS3Period"=0, "LS3PulseWidth"=0, "LS4Period"=0, "LS4PulseWidth"=0} ("LowsidePWM"), "LS1Period"=w282, "LS1PulseWidth"=w283, "LS2Period"=w284, "LS2PulseWidth"=w285, "LS3Period"=w286, "LS3PulseWidth"=w287, "LS4Period"=w288, "LS4PulseWidth"=w289) -> (w248:T25)
    n115 = call <vilib>:"pfi_rt_control_revg2.vi"("PFIControl"="PFIControl") -> ("PFIControlToFPGA"=w249:T28)  [unwired: 4 in]
    n116 = xnode "Read/Write Control"("FPGA VI Reference In"=w244, "PFIControl"=w249, "LowsidePWM"=w248, "PFI_IPhaseInterface"=w246) -> ("FPGA VI Reference Out"=w272:refnum<k20>)  [unwired: 1 in, 1 out]
    n117 = local read "Stroke (FALSE=2, TRUE=4)"() -> (w268:bool)
    n118 = local read "MAX_CAT"() -> (w269:u16)
    n119 = call <vilib>:"Offset2CAT.vi"("Offset (CAD Before TDC)"="FuelTiming (DBTDC)", "TDC (Absolute CAD)"="TDC1", "MAX_CAT"=w269, "Stroke (FALSE=2, TRUE=4)"=w268) -> ("CAT"=w254:u16)  [unwired: 1 out]
    n120 = call <vilib>:"Offset2CAT.vi"("Offset (CAD Before TDC)"="CutoffPosition (DBTDC)", "TDC (Absolute CAD)"="TDC1", "MAX_CAT"=w269, "Stroke (FALSE=2, TRUE=4)"=w268) -> ("CAT"=w255:u16)  [unwired: 1 out]
    n121 = call <vilib>:"time2ticks.vi"("Time (msec)"="PFIDuration") -> ("Ticks"=w256:u32)  [unwired: 1 in]
    n122 = call <vilib>:"Offset2CAT.vi"("Offset (CAD Before TDC)"="FuelTiming (DBTDC)", "TDC (Absolute CAD)"="TDC2", "MAX_CAT"=w269, "Stroke (FALSE=2, TRUE=4)"=w268) -> ("CAT"=w258:u16)  [unwired: 1 out]
    n123 = call <vilib>:"Offset2CAT.vi"("Offset (CAD Before TDC)"="CutoffPosition (DBTDC)", "TDC (Absolute CAD)"="TDC2", "MAX_CAT"=w269, "Stroke (FALSE=2, TRUE=4)"=w268) -> ("CAT"=w259:u16)  [unwired: 1 out]
    n124 = call <vilib>:"time2ticks.vi"("Time (msec)"="PFIDuration") -> ("Ticks"=w260:u32)  [unwired: 1 in]
    n125 = Bundle By Name(cluster=w266, "FuelEnable"="FuelEnable1", "PositionMode"=TRUE, "ActiveLow"=FALSE, "StartPosition"=w254, "CutoffPosition"=w255, "Duration"=w256) -> (w250:T17)
    n126 = Bundle By Name(cluster=w266, "FuelEnable"="FuelEnable2", "PositionMode"=TRUE, "ActiveLow"=FALSE, "StartPosition"=w258, "CutoffPosition"=w259, "Duration"=w260) -> (w265:T17)
    n127 = xnode "Read/Write Control"("FPGA VI Reference In"=w272, "FuelControl1"=w250, "FuelControl2"=w265) -> ()  [unwired: 1 in, 2 out]
    n128 = node-c288() -> ()  [unwired: 1 in, 1 out]
  }
  n129 = node-c288(w8) -> ()
  n130 = xnode "Close FPGA VI Reference"("FPGA VI Reference In"=w7) -> ()  [unwired: 1 in, 1 out]
  n131 = node-c288(w5) -> ()  [unwired: 1 out]
  n132 = node-c288(w3) -> ()  [unwired: 1 out]
